vi "ReadDataQueue.vi"(7 "Write/nRead":bool, 8 "error in (no error)":errorcluster, 11 "Output Waveform":u16[](array[numeric])) -> (0 "error out":errorcluster, 3 "WaveOut":i16[](array[numeric]))   [LabVIEW 2020]
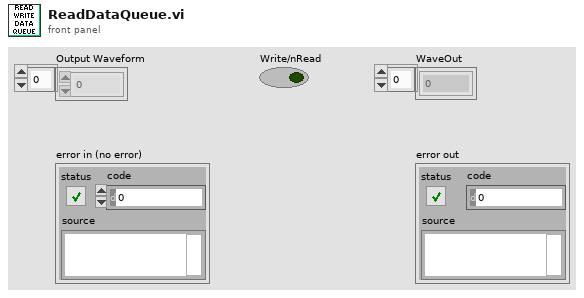
[diagram p1: front panel]
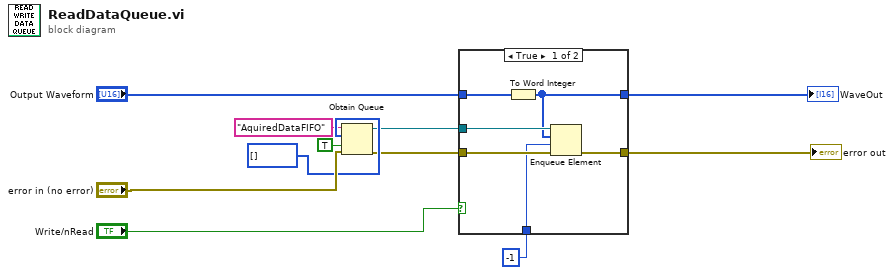
[diagram p0: block diagram]
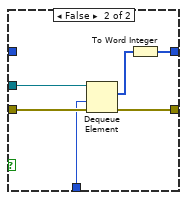
[diagram p2: hidden frame]
diagram:
  n1 = Obtain Queue(name (unnamed)="AquiredDataFIFO", element data type=i16[] [] ("16bit integer"), create if not found? (T)=TRUE, error in (no error)="error in (no error)") -> (queue out=w3:refnum<queue>, error out=w2:errorcluster)  [unwired: 1 in, 1 out]
  n2 = case shown="True" "Write/nRead" {
    tunnel: "Output Waveform" -> [w17 _]
    tunnel: [w16 w23] -> w10
    tunnel: w3 -> [w15 w22]
    tunnel: w2 -> [w14 w21]
    tunnel: -1 -> [w13 w20]
    tunnel: [w12 w18] -> w7
    frame True {
      n3 = To Word Integer(number=w17) -> (16bit integer=w12:i16[])
      n4 = Enqueue Element(queue=w15, element=w12, timeout in ms (-1)=w13, error in (no error)=w14) -> (error out=w16:errorcluster)  [unwired: 2 out]
    }
    frame False {
      n5 = Dequeue Element(queue=w22, timeout in ms (-1)=w20, error in (no error)=w21) -> (element=w19:i16[], error out=w23:errorcluster)  [unwired: 2 out]
      n6 = To Word Integer(number=w19) -> (16bit integer=w18:i16[])
    }
  }
  "error out" <- w10
  "WaveOut" <- w7
